vi "VALID RFID.vi"(5 "Tag Change":bool=TRUE, 6 "Cycle Start":bool, 7 "Bypass?":bool=TRUE, 9 "RFID-1":string, 10 "RFID":string) -> (1 "RFID OUT":string, 2 "CHANGED?":bool)   [LabVIEW 2020]
panel:
  out "VALID?":bool
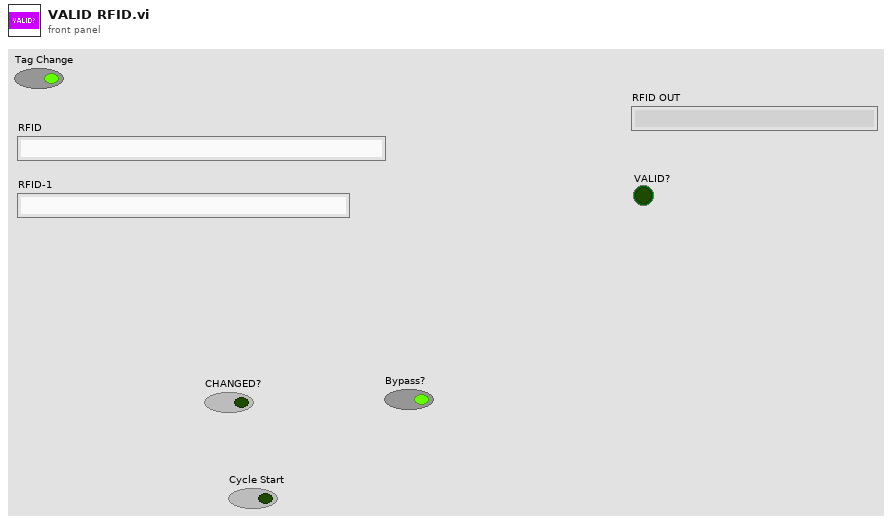
[diagram p1: front panel]
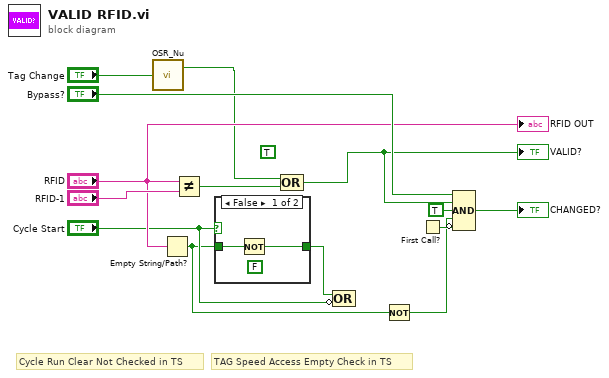
[diagram p0: block diagram]
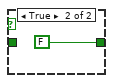
[diagram p2: hidden frame]
diagram:
  (unwired) TRUE ("result")
  # "TAG Speed Access Empty Check in TS"
  # "Cycle Run Clear Not Checked in TS"
  n1 = call "OSR_Nu.vi"("input"="Tag Change") -> ("Rising"=w7:bool)  [unwired: 3 in, 1 out]
  n2 = Empty String/Path?(string/path="RFID") -> (empty?=w2:bool)
  n3 = Not Equal?(x="RFID", y="RFID-1") -> (x != y?=w14:bool)
  n4 = case shown="False" "Cycle Start" {
    tunnel: w2 -> [w16 _]
    tunnel: [w15 FALSE] -> w6
    frame False {
      (unwired) FALSE
      n5 = Not(x=w16) -> (.not. x?=w15:bool)
    }
    frame True {
    }
  }
  n6 = Compound Arithmetic op=OR(w7, w14) -> (w3:bool)
  "VALID?" <- w3
  n7 = Compound Arithmetic op=OR(w6, invert "Cycle Start") -> ()  [unwired: 1 out]
  n8 = Not(x=w2) -> (.not. x?=w1:bool)
  n9 = First Call?() -> (First Call?: T/F=w8:bool)
  n10 = Compound Arithmetic op=AND("Bypass?", w3, TRUE ("value"), w1, invert w8) -> (→"CHANGED?":bool)
  "RFID OUT" <- "RFID"
